vi "Sort Ancestors.vi"(8 "error in (no error)":errorcluster, 11 "Classes":refnum<class>[](array[class])) -> (0 "error out":errorcluster, 3 "Sorted Classes":refnum<class>[](array[class]))   [LabVIEW 2017, in "Composition.lvlib"]
doc: "Sorts classes from last child to eldest parent."
uses:
  Composition.lvlib
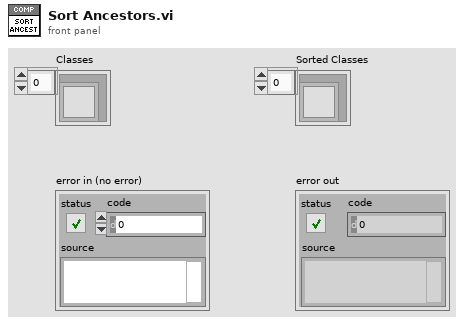
[diagram p1: front panel]
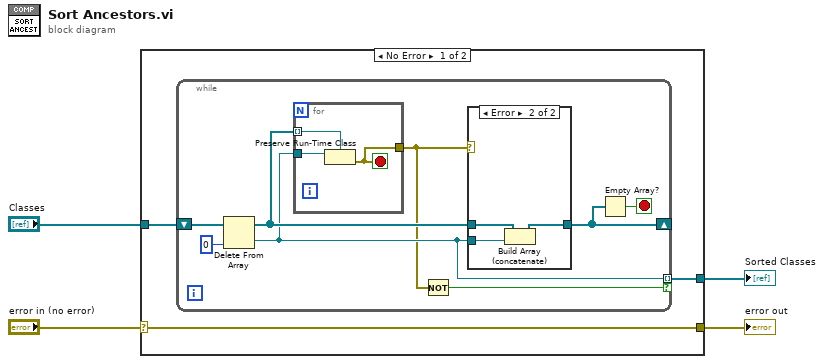
[diagram p0: block diagram]
diagram:
  n1 = case shown="No Error" "error in (no error)" {
    selector: "error in (no error)" -> [w5 w23]
    tunnel: "Classes" -> [w7 _]
    tunnel: [w6 _] -> w3
    tunnel: [w5 w23] -> w1
    frame No Error {
      n2 = while {
        shift-right: [w10] -> _
        shift-left: w7 -> [w15]
        tunnel: [w11] -> w6 mode=indexing if=w9
        stop <- w13 stop-if-true
        n3 = Delete From Array(array=w15, index=0) -> (deleted portion=w11:refnum<class>, array with subset deleted=w12:refnum<class>[])  [unwired: 1 in]
        n4 = for {
          tunnel: w11 -> [w22]
          tunnel: w12 -> [w21] mode=indexing
          tunnel: [w20] -> w8
          stop <- w20 stop-if-true
          n5 = Preserve Run-Time Class(object in=w22, 2:w21) -> (error out=w20:errorcluster)  [unwired: 1 in, 1 out]
        }
        n6 = Not(x=w8) -> (.not. x?=w9:bool)
        n7 = case shown="Error" w8 {
          tunnel: w12 -> [w16 w19]
          tunnel: [w16 w18] -> w10
          tunnel: w11 -> [_ w17]
          frame No Error {
          }
          frame Error {
            n8 = Build Array (concatenate)(w19, w17) -> (w18:refnum<class>[])
          }
        }
        n9 = Empty Array?(array=w10) -> (empty?=w13:bool)
      }
    }
    frame Error {
    }
  }
  "Sorted Classes" <- w3
  "error out" <- w1
